vi "New File (4-28-20220) v2.vi"() -> ()   [LabVIEW 2020]
panel:
  in  "message":string="New file created on 4-28-2022 v2"
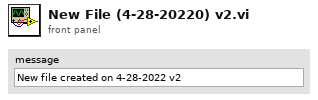
[diagram p1: front panel]
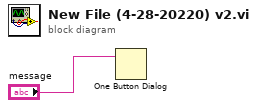
[diagram p0: block diagram]
diagram:
  n1 = One Button Dialog(message="message") -> ()  [unwired: 1 in, 1 out]
